vi "Clean.vi"(7 "bulid type":T1, 8 "error in (no error)":errorcluster, 11 "package builder solution path":path) -> (0 "error out":errorcluster)   [LabVIEW 2021, in "NI Package Builder API.lvlib"]
uses:
  build type.ctl
  NI Package Builder API.lvlib
panel:
  out "command line standard output":string
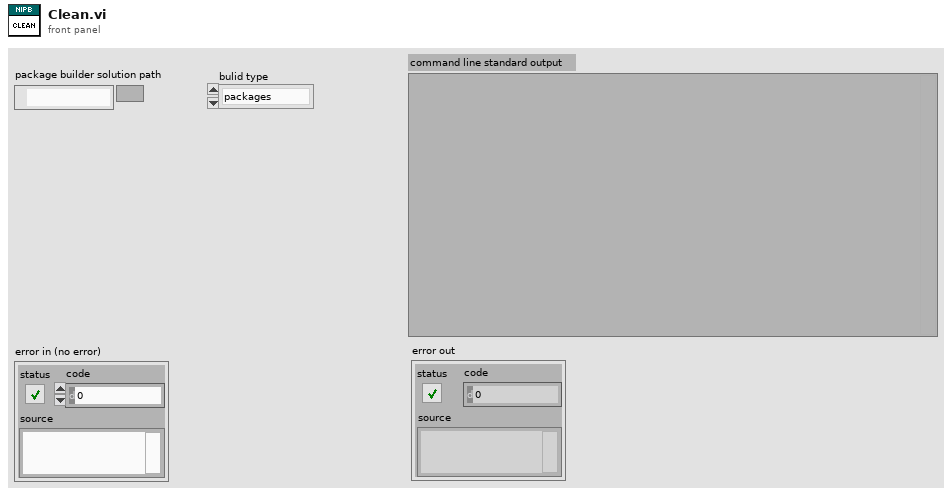
[diagram p1: front panel]
types:
  T1 = typedef "NI Package Builder API.lvlib/build type.ctl" = enum16{"packages", "feeds", "solution"}
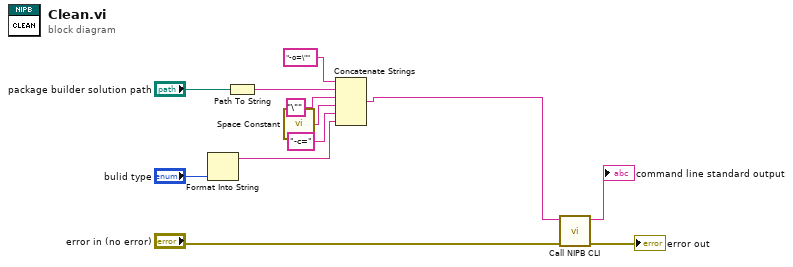
[diagram p0: block diagram]
diagram:
  n1 = Format Into String("bulid type") -> (resulting string=w5:string)  [unwired: 3 in, 1 out]
  n2 = Path To String(path="package builder solution path") -> (string=w8:string)
  n3 = call <vilib>:"Space Constant.vi"() -> ("String"=w4:string)
  n4 = Concatenate Strings("-o=\"" ("string"), w8, "\"", w4, "-c=" ("string"), w5) -> (w1:string)
  n5 = call "Call NIPB CLI.vi"("error in (no error)"="error in (no error)", "command"=w1) -> ("error out"=→"error out":errorcluster, "command line standard output"=→"command line standard output":string)  [unwired: 8 in]
